vi "UnloadAction.vi"(8 "error in (no error)":errorcluster caption="entrée d'erreur (pas d'erreur)", 11 "OR77200 en entrée":refnum<class "EG_G5210.lvclass"> caption="DNL_LabVIEW Object in") -> (0 "error out":errorcluster caption="sortie d'erreur", 3 "OR77200 en sortie":refnum<class "EG_G5210.lvclass"> caption="DNL_LabVIEW Object out")   [LabVIEW 2010, in "EG_G5210.lvclass"]
uses:
  EG_G5210.lvclass
  BaseDevice/BaseDevice.lvclass
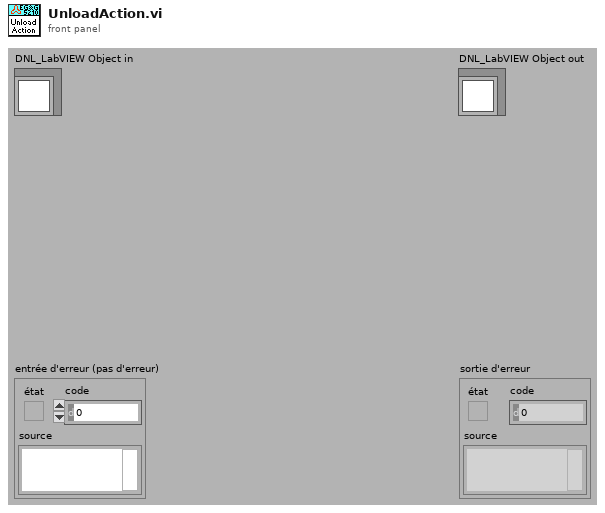
[diagram p1: front panel]
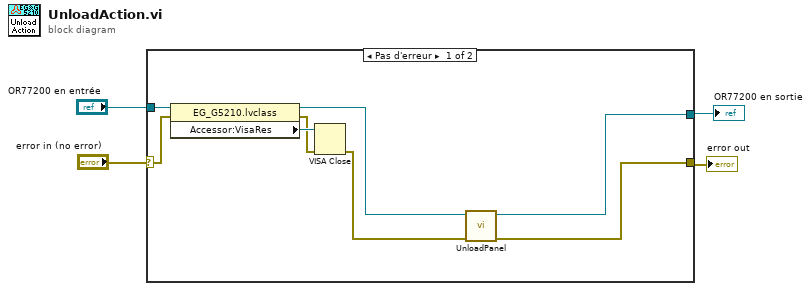
[diagram p0: block diagram]
diagram:
  n1 = case shown="Pas d'erreur" "error in (no error)" {
    selector: "error in (no error)" -> [w6 w13]
    tunnel: [w8 w13] -> w3
    tunnel: [w7 w14] -> w2
    tunnel: "OR77200 en entrée" -> [w12 w14]
    frame No Error {
      n2 = property class="EG_G5210.lvclass"(reference=w12, error in=w6) -> (reference out=w9:refnum<class "EG_G5210.lvclass">, error out=w5:errorcluster, "Accessor:VisaRes"=w11:refnum<visa-resource-name>)
      n3 = VISA Close(VISA resource name=w11, error in (no error)=w5) -> (error out=w10:errorcluster)
      n4 = call "UnloadPanel.vi"("error in (no error)"=w10, "Device en entrée"=w9) -> ("error out"=w8:errorcluster, "Device en sortie"=w7:refnum<class "EG_G5210.lvclass">)  [unwired: 8 in]
    }
    frame Error {
    }
  }
  "error out" <- w3
  "OR77200 en sortie" <- w2
